vi "sort-pannel-list.vi"(11 "sce-pannel-list":T1(array[cluster]) {"pannel"."ID" format="%02x"}) -> (3 "sorted-sce-pannel-list":T1(array[cluster]))   [LabVIEW 2019]
panel:
  in  "模式列表":T2(array[cluster]) {"sce-pannel-list"."pannel"."ID" format="%02x"}
  out "已排序的数组":dbl[](array[numeric])
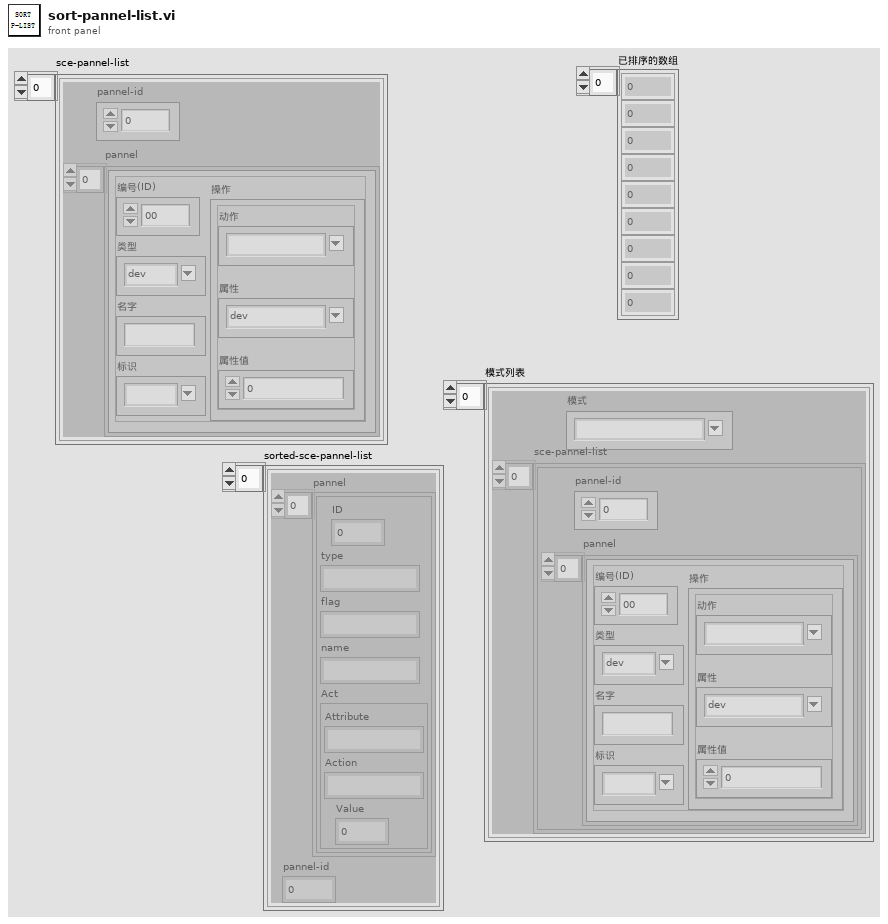
[diagram p1: front panel]
types:
  T1 = cluster{"pannel":cluster{"ID":u8, "type":string, "flag":string, "name":string, "Act":cluster{"Attribute":string, "Action":string, "Value":dbl}}[], "pannel-id":dbl}[]
  T2 = cluster{"模式":string, "sce-pannel-list":cluster{"pannel":cluster{"ID":u8, "type":string, "flag":string, "name":string, "Act":cluster{"Attribute":string, "Action":string, "Value":dbl}}[], "pannel-id":dbl}[]}[]
  T3 = cluster{"pannel":cluster{"ID":u8, "type":string, "flag":string, "name":string, "Act":cluster{"Attribute":string, "Action":string, "Value":dbl}}[], "pannel-id":dbl}
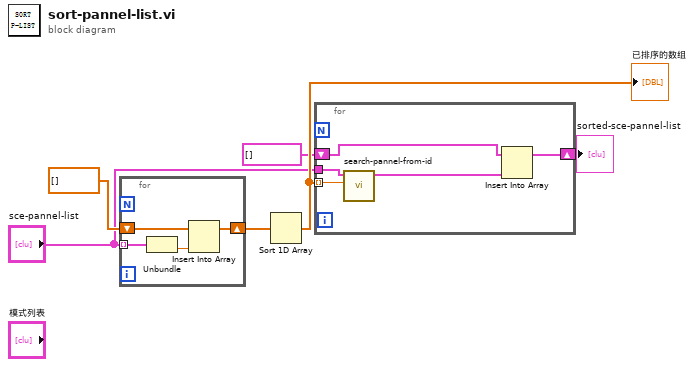
[diagram p0: block diagram]
diagram:
  n1 = for {
    tunnel: "sce-pannel-list" -> [w10] mode=indexing
    shift-right: [w8] -> w5
    shift-left: dbl[] [] -> [w7]
    n2 = Unbundle(w10) -> ("pannel-id"=w9:dbl)  [unwired: 1 out]
    n3 = Insert Into Array(array=w7, new element=w9) -> (w8:dbl[])  [unwired: 1 in]
  }
  n4 = Sort 1D Array(array=w5) -> (sorted array=w4:dbl[])
  "已排序的数组" <- w4
  n5 = for {
    tunnel: w4 -> [w14] mode=indexing
    tunnel: "sce-pannel-list" -> [w15]
    shift-right: [w12] -> w1
    shift-left: T1 [] -> [w11]
    n6 = call "search-pannel-from-id.vi"("pannel-id"=w14, "sce-pannel-list"=w15) -> ("sce-pannel"=w13:T3)  [unwired: 9 in]
    n7 = Insert Into Array(array=w11, new element=w13) -> (w12:T1)  [unwired: 1 in]
  }
  "sorted-sce-pannel-list" <- w1
